vi "OSW - 64bit - Sample.vi"() -> ()   [LabVIEW 2013]
uses:
  <vilib>/Instr/_visa.llb/VISA Configure Serial Port (Instr).vi
panel:
  in  "Switch state":bool
  in  "Stop program":bool
  out "OSW model":string
  in  "VISA resource name":refnum<visa-resource-name>
  # "State 2\nCross State"
  # "State 1\nBar State"
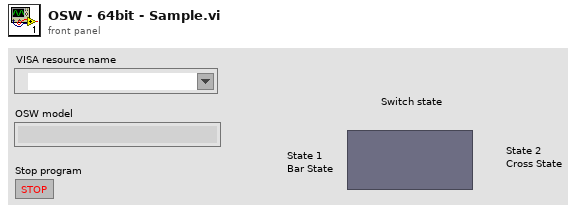
[diagram p1: front panel]
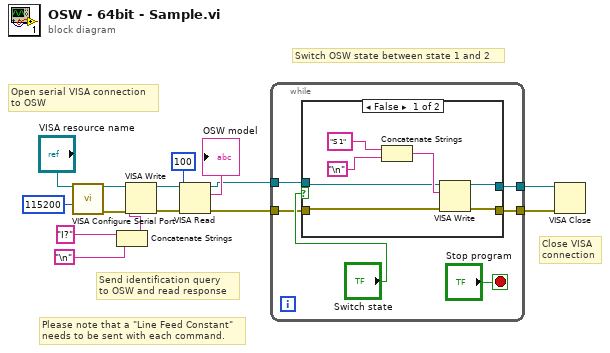
[diagram p0: block diagram]
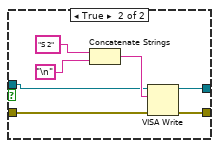
[diagram p2: hidden frame]
diagram:
  # "Please note that a \"Line Feed Constant\"\nneeds to be sent with each command."
  # "Close VISA\nconnection"
  # "Send identification query\nto OSW and read response"
  # "Open serial VISA connection\nto OSW"
  # "Switch OSW state between state 1 and 2"
  n1 = call-poly "VISA Configure Serial Port"("VISA resource name"="VISA resource name", "baud rate (9600)"=u32 115200) -> ("VISA resource name out"=w6:refnum<visa-resource-name>, "error out"=w5:errorcluster)  [unwired: 12 in]
  n2 = Concatenate Strings("I?" ("String 2"), "\n") -> (w11:string)
  n3 = VISA Write(VISA resource name=w6, write buffer=w11, error in (no error)=w5) -> (VISA resource name out=w10:refnum<visa-resource-name>, error out=w9:errorcluster)  [unwired: 1 out]
  n4 = VISA Read(VISA resource name=w10, byte count=u32 100, error in (no error)=w9) -> (VISA resource name out=w3:refnum<visa-resource-name>, read buffer=→"OSW model":string, error out=w4:errorcluster)  [unwired: 1 out]
  n5 = while {
    tunnel: w4 -> [w19]
    tunnel: w3 -> [w18]
    tunnel: [w17] -> w2
    tunnel: [w16] -> w1
    stop <- "Stop program" stop-if-true
    n6 = case shown="False" "Switch state" {
      tunnel: w19 -> [w23 w32]
      tunnel: w18 -> [w22 w31]
      tunnel: [w25 w30] -> w17
      tunnel: [w24 w29] -> w16
      frame False {
        n7 = Concatenate Strings("S 1" ("String"), "\n") -> (w28:string)
        n8 = VISA Write(VISA resource name=w22, write buffer=w28, error in (no error)=w23) -> (VISA resource name out=w25:refnum<visa-resource-name>, error out=w24:errorcluster)  [unwired: 1 out]
      }
      frame True {
        n9 = Concatenate Strings("S 2" ("String"), "\n") -> (w35:string)
        n10 = VISA Write(VISA resource name=w31, write buffer=w35, error in (no error)=w32) -> (VISA resource name out=w30:refnum<visa-resource-name>, error out=w29:errorcluster)  [unwired: 1 out]
      }
    }
  }
  n11 = VISA Close(VISA resource name=w2, error in (no error)=w1) -> ()  [unwired: 1 out]
